vi "OCR_Select and Look for Char.vi"(4 "Ambiguous\nat Beginning":bool, 6 "Ambiguous\nat End":bool, 7 "Color Set":T1, 8 "Error":errorcluster, 9 "Index":i16, 10 "Width":i32, 11 "2D Image":u32[][](array[colorbox])) -> (0 "Error Out":errorcluster, 3 "Char Out":T2)   [LabVIEW 2009]
uses:
  Controls/String_Picture/String Char Normal.ctl
  Controls/Cluster/Cluster_Text Color Set.ctl
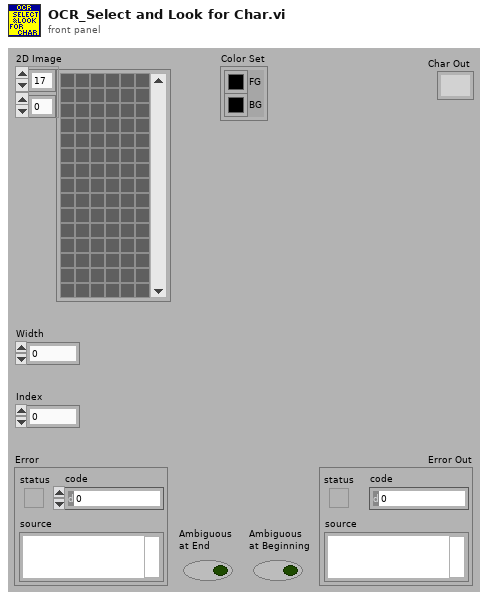
[diagram p1: front panel]
types:
  T1 = typedef "Cluster_Text Color Set.ctl" = cluster{"BG":u32, "FG":u32}
  T2 = typedef "String Char Normal.ctl" = string
  T3 = typedef "Array Bool Char Bits Wide.ctl" = bool[][]
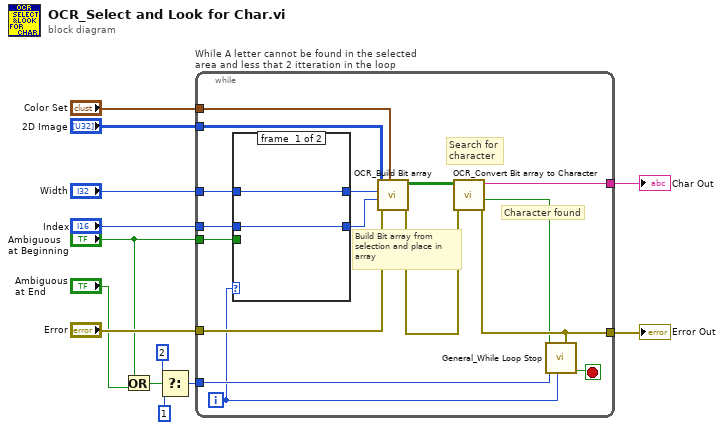
[diagram p0: block diagram]
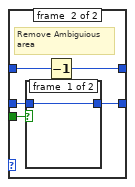
[diagram p2: hidden frame]
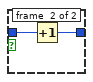
[diagram p3: hidden frame]
diagram:
  n1 = Or(x="Ambiguous\nat Beginning", y="Ambiguous\nat End") -> (x .or. y?=w5:bool)
  n2 = Select(t=2 ("Array Size In"), s=w5, f=1 ("Array Size In")) -> (s? t:f=w4:i32)
  n3 = while "While A letter cannot be found in the selected area and less that 2 itteration in the loop" {
    tunnel: [w28] -> w13
    tunnel: [w23] -> w12
    tunnel: "Index" -> [w18]
    tunnel: "Width" -> [w19]
    tunnel: "Error" -> [w26]
    tunnel: "Color Set" -> [w25]
    tunnel: "2D Image" -> [w24]
    tunnel: w4 -> [w21]
    tunnel: "Ambiguous\nat Beginning" -> [w17]
    i -> [w20]
    stop <- w22 stop-if-true
    # "Search for \ncharacter"
    # "Build Bit array from\nselection and place in \narray"
    # "Character found"
    n4 = case shown="..0" w20 {
      tunnel: w19 -> [w31 w35]
      tunnel: w18 -> [w30 w33]
      tunnel: w17 -> [_ w36]
      tunnel: [w31 w34] -> w16
      tunnel: [w30 w32] -> w15
      frame #0 {
      }
      frame #1 {
        # "Remove Ambiguious\narea"
        n5 = case shown="True" w36 {
          tunnel: w33 -> [w37 w39]
          tunnel: [w37 w38] -> w32
          frame #0 {
          }
          frame #1 {
            n6 = Increment(x=w39) -> (x+1=w38:i16)
          }
        }
        n7 = Decrement(x=w35) -> (x-1=w34:i32)
      }
    }
    n8 = call "OCR_Build Bit array.vi"("Color Set"=w25, "Error"=w26, "Index"=w15, "Width"=w16, "2D Image"=w24) -> ("Error Out"=w27:errorcluster, "Bit Array Out"=w29:T3)  [unwired: 5 in]
    n9 = call "OCR_Convert Bit array to Character.vi"("Error"=w27, "Bit Array"=w29) -> ("Error Out"=w23:errorcluster, "Found Out"=w14:bool, "Char Out"=w28:T2)  [unwired: 7 in]
    n10 = call "General_While Loop Stop.vi"("Error In"=w23, "Index In"=w20, "Array Size In"=w21, "Stop 1 In"=w14) -> ("Stop Out3"=w22:bool)  [unwired: 3 in, 3 out]
  }
  "Char Out" <- w13
  "Error Out" <- w12
